vi "Shift Registers.vi"() -> ()   [LabVIEW 2019]
panel:
  out "Previous Number":dbl
  in  "stop":bool
  out "Random Number":dbl
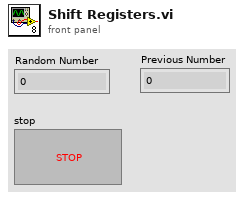
[diagram p1: front panel]
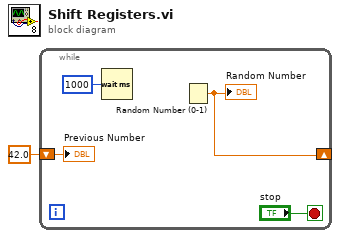
[diagram p0: block diagram]
diagram:
  n1 = while {
    shift-right: [w3] -> _
    shift-left: 42.0 ("number: 0 to 1") -> [w2]
    stop <- "stop" stop-if-true
    n2 = Wait (ms)(milliseconds to wait=u32 1000) -> ()  [unwired: 1 out]
    n3 = Random Number (0-1)() -> (number: 0 to 1=w3:dbl)
    "Random Number" <- w3
    "Previous Number" <- w2
  }
